vi "PH_SRDG645.PC Write PSDB.vi"(0 "i ref in":refnum<vi>, 5 "error IO":errorcluster) -> (14 "i ref out":refnum<vi>, 19 "error out":errorcluster)   [LabVIEW 2014, in "PH_SRDG645.lvlib"]
doc: "This is the proc case which writes data to the PHELIX shot data base."
uses:
  PH_SRDG645.lvlib
  PH_Basics/PH_PSDBWriter/PH_PSDBWriter.Numeric dataset.ctl
  PH_Basics/PH_PSDBWriter/PH_PSDBWriter.lvlib
  PH_Basics/PH_StatusHandler/PH_StatusHandler.lvlib
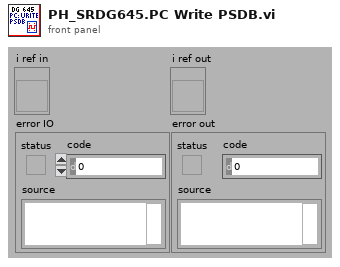
[diagram p1: front panel]
types:
  T1 = typedef "PH_PSDBWriter.lvlib/PH_PSDBWriter.Numeric dataset.ctl" = cluster{"name":string, "data":dbl, "unit":string}
  T2 = typedef "PH_SRDG645.lvlib/PH_SRDG645.i attribute.ctl" = cluster{"GUI Refs":cluster{"Delete":refnum<vi>, "Device Errors":refnum<vi>, "Trigger":refnum<vi>, "Default Name":refnum<vi>, "Firmware Revision":refnum<vi>, "Serial Number":refnum<vi>, "Model":refnum<vi>, "Visa resource name":refnum<vi>}, "Service ID Rate":i32, "Service IDs Channelinfo":i32[], "VISA resource name":refnum<visa-resource-name>, "Device Errors":cluster{"code":i32, "Text":string}[], "Trigger":T3, "Channels":cluster{"T1":T4, "A":T4, "B":T4, "C":T4, "D":T4, "E":T4, "F":T4, "G":T4, "H":T4}, "GUI Refs Channels":refnum<vi>[], "Outputs":cluster{"AB":cluster{"Level Offset [V]":dbl, "Amplitue [V]":dbl, "Polarity":i32}, "CD":cluster{"Level Offset [V]":dbl, "Amplitue [V]":dbl, "Polarity":i32}, "EF":cluster{"Level Offset [V]":dbl, "Amplitue [V]":dbl, "Polarity":i32}, "GH":cluster{"Level Offset [V]":dbl, "Amplitue [V]":dbl, "Polarity":i32}, "T0":cluster{"Level Offset [V]":dbl, "Amplitue [V]":dbl, "Polarity":i32}}, "GUI Refs Outputs":refnum<vi>[], "Serial Number":string, "Firmweare Revision":string, "Model":string}
  T3 = typedef "PH_SRDG645.lvlib/PH_SRDG645.Trigger.ctl" = cluster{"Source":i32, "Rate [Hz]":dbl, "Level [V]":dbl}
  T4 = typedef "PH_SRDG645.lvlib/PH_SRDG645.Channel Settings.ctl" = cluster{"Delay [s]":dbl, "relative to":i32}
  T5 = cluster{"Level Offset [V]":dbl, "Amplitue [V]":dbl, "Polarity":i32}
  T6 = cluster{"Level Offset [V]":dbl, "Amplitue [V]":dbl, "Polarity":i32}[]
  T7 = typedef "PH_PSDBWriter.lvlib/PH_PSDBWriter.String dataset.ctl" = cluster{"name":string, "data":string, "unit":string}
  T8 = typedef "PH_PSDBWriter.lvlib/PH_PSDBWriter.PSDB Dataset.ctl" = cluster{"Version":i32, "2D data Input":T9[], "Boolean Input":T11[], "Image Input":T12[], "Numeric Input":T1[], "String Input":T7[]}
  T9 = typedef "PH_PSDBWriter.lvlib/PH_PSDBWriter.2D dataset.ctl" = cluster{"name":string, "data":dbl[][], "axis description":T10}
  T10 = typedef "PSDB.lvlib/PSDB_AxisDescription.ctl" = cluster{"x axis label":string, "y axis label":string, "x axis unit":string, "y axis unit":string}
  T11 = typedef "PH_PSDBWriter.lvlib/PH_PSDBWriter.Boolean dataset.ctl" = cluster{"name":string, "data":bool, "unit":string}
  T12 = typedef "PH_PSDBWriter.lvlib/PH_PSDBWriter.Image dataset.ctl" = cluster{"name":string, "data":T13, "unit":string}
  T13 = typedef "IMAQ Image.ctl" = refnum<image>
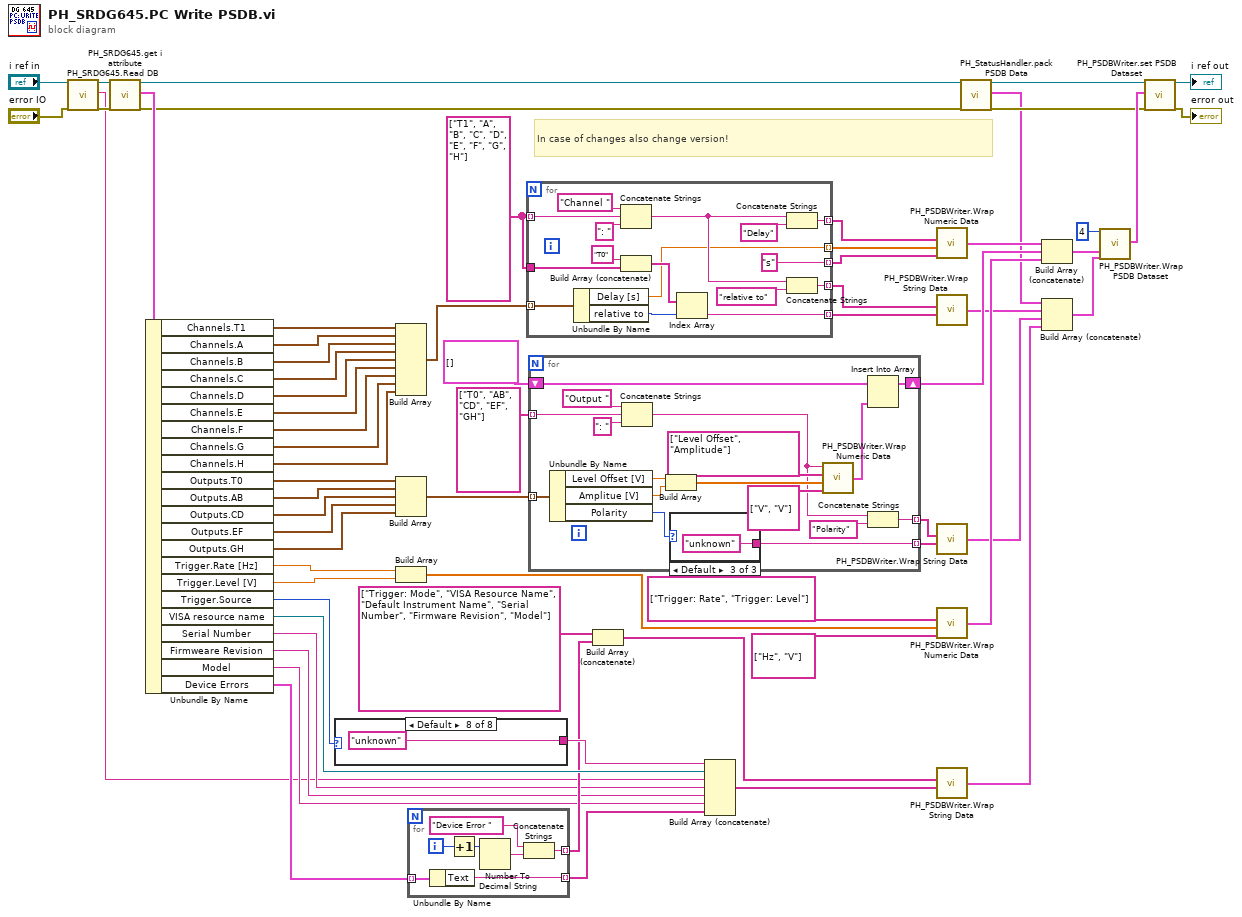
[diagram p0: block diagram]
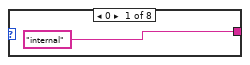
[diagram p2: hidden frame]
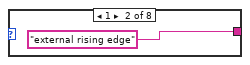
[diagram p3: hidden frame]
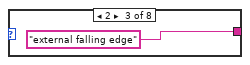
[diagram p4: hidden frame]
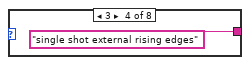
[diagram p5: hidden frame]
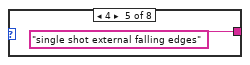
[diagram p6: hidden frame]
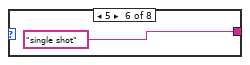
[diagram p7: hidden frame]
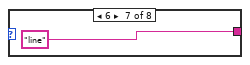
[diagram p8: hidden frame]
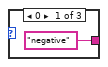
[diagram p9: hidden frame]
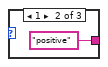
[diagram p10: hidden frame]
diagram:
  w32 = string[] ["T1", "A", "B", "C", "D", "E", "F", "G", "H"]
  # "In case of changes also change version!"
  n1 = call "PH_SRDG645.Read DB.vi"("i ref in"="i ref in", "error in"="error IO") -> ("i ref out"=w15:refnum<vi>, "Default Name"=w14:string, "error out"=w16:errorcluster)  [unwired: 15 in]
  n2 = call "PH_SRDG645.get i attribute.vi"("i ref in"=w15, "error in (no error)"=w16) -> ("i ref out"=w4:refnum<vi>, "i attribute"=w49:T2, "error out"=w5:errorcluster)  [unwired: 15 in]
  n3 = Unbundle By Name(w49) -> ("Channels.T1"=w66:T4, "Channels.A"=w65:T4, "Channels.B"=w64:T4, "Channels.C"=w63:T4, "Channels.D"=w62:T4, "Channels.E"=w37:T4, "Channels.F"=w61:T4, "Channels.G"=w36:T4, "Channels.H"=w35:T4, "Outputs.T0"=w60:T5, "Outputs.AB"=w59:T5, "Outputs.CD"=w58:T5, "Outputs.EF"=w57:T5, "Outputs.GH"=w38:T5, "Trigger.Rate [Hz]"=w42:dbl, "Trigger.Level [V]"=w55:dbl, "Trigger.Source"=w47:i32, "VISA resource name"=w52:refnum<visa-resource-name>, "Serial Number"=w19:string, "Firmweare Revision"=w18:string, "Model"=w17:string, "Device Errors"=w53:cluster{"code":i32, "Text":string}[])
  n4 = case shown="Default" w47 {
    tunnel: ["internal" "external rising edge" "external falling edge" "single shot external rising edges" "single shot external falling edges" "single shot" "line" "unknown"] -> w46
    frame 0 {
    }
    frame 1 {
    }
    frame 2 {
    }
    frame 3 {
    }
    frame 4 {
    }
    frame 5 {
    }
    frame 6 {
    }
    frame Default {
    }
  }
  n5 = Build Array(w66, w65, w64, w63, w62, w37, w61, w36, w35) -> (w26:T4[])
  n6 = Build Array(w60, w59, w58, w57, w38) -> (w56:T6)
  n7 = Build Array(w42, w55) -> (w41:dbl[])
  n8 = for {
    tunnel: w53 -> [w81] mode=indexing
    tunnel: [w80] -> w51 mode=indexing
    tunnel: [w75] -> w44 mode=indexing
    i -> [w79]
    n9 = Unbundle By Name(w81) -> ("Text"=w80:string)
    n10 = Increment(x=w79) -> (x+1=w78:i32)
    n11 = Number To Decimal String(number=w78) -> (decimal integer string=w76:string)  [unwired: 1 in]
    n12 = Concatenate Strings("Device Error ", w76) -> (w75:string)
  }
  n13 = for {
    tunnel: w26 -> [w97] mode=indexing
    tunnel: w32 -> [w94] mode=indexing
    tunnel: w32 -> [w93]
    tunnel: [w89] -> w31 mode=indexing
    tunnel: [w87] -> w30 mode=indexing
    tunnel: ["s" ("string")] -> w28 mode=indexing
    tunnel: [w83] -> w27 mode=indexing
    tunnel: [w82] -> w29 mode=indexing
    n14 = Unbundle By Name(w97) -> ("Delay [s]"=w82:dbl, "relative to"=w90:i32)
    n15 = Concatenate Strings("Channel ", w94, ": " ("string")) -> (w85:string)
    n16 = Build Array (concatenate)("T0", w93) -> (w91:string[])
    n17 = Index Array(array=w91, index=w90) -> (element=w89:string)
    n18 = Concatenate Strings(w85, "Delay" ("string")) -> (w83:string)
    n19 = Concatenate Strings(w85, "relative to" ("string")) -> (w87:string)
  }
  n20 = for {
    tunnel: w56 -> [w114] mode=indexing
    shift-right: [w113] -> w24
    shift-left: T1[] [] -> [w112]
    tunnel: string[] ["T0", "AB", "CD", "EF", "GH"] -> [w106] mode=indexing
    tunnel: [w101] -> w34 mode=indexing
    tunnel: [w98] -> w33 mode=indexing
    n21 = Unbundle By Name(w114) -> ("Level Offset [V]"=w107:dbl, "Amplitue [V]"=w108:dbl, "Polarity"=w102:i32)
    n22 = Concatenate Strings("Output " ("string"), w106, ": " ("string")) -> (w100:string)
    n23 = Build Array(w107, w108) -> (w105:dbl[])
    n24 = case shown="Default" w102 {
      tunnel: ["negative" ("string") "positive" ("string") "unknown" ("string")] -> w101
      frame 0 {
      }
      frame 1 {
      }
      frame Default {
      }
    }
    n25 = call "PH_PSDBWriter.Wrap Numeric Data.vi"("Unit Array"=string[] ["V", "V"], "Data Array"=w105, "Name Array"=string[] ["Level Offset", "Amplitude"], "Name Prefix"=w100) -> ("PSDB Numeric Data Array"=w109:T1[])
    n26 = Insert Into Array(array=w112, new element=w109) -> (w113:T1[])  [unwired: 1 in]
    n27 = Concatenate Strings(w100, "Polarity") -> (w98:string)
  }
  n28 = Build Array (concatenate)(string[] ["Trigger: Mode", "VISA Resource Name", "Default Instrument Name", "Serial Number", "Firmware Revision", "Model"], w44) -> (w43:string[])
  n29 = Build Array (concatenate)(w46, w52, w14, w19, w18, w17, w51) -> (w48:string[])
  n30 = call "PH_PSDBWriter.Wrap Numeric Data.vi"("Unit Array"=w28, "Data Array"=w29, "Name Array"=w27) -> ("PSDB Numeric Data Array"=w25:T1[])  [unwired: 1 in]
  n31 = call "PH_PSDBWriter.Wrap String Data.vi"("Data Array"=w31, "Name Array"=w30) -> ("PSDB String Data Array"=w22:T7[])  [unwired: 2 in]
  n32 = call "PH_PSDBWriter.Wrap String Data.vi"("Data Array"=w34, "Name Array"=w33) -> ("PSDB String Data Array"=w21:T7[])  [unwired: 2 in]
  n33 = call "PH_PSDBWriter.Wrap Numeric Data.vi"("Unit Array"=string[] ["Hz", "V"], "Data Array"=w41, "Name Array"=string[] ["Trigger: Rate", "Trigger: Level"]) -> ("PSDB Numeric Data Array"=w23:T1[])  [unwired: 1 in]
  n34 = call "PH_PSDBWriter.Wrap String Data.vi"("Data Array"=w48, "Name Array"=w43) -> ("PSDB String Data Array"=w20:T7[])  [unwired: 2 in]
  n35 = call "PH_StatusHandler.pack PSDB Data.vi"("VI in"=w4, "error in (no error)"=w5) -> ("VI out"=w2:refnum<vi>, "PSDB String Data Array"=w1:T7[], "error out"=w3:errorcluster)  [unwired: 15 in]
  n36 = Build Array (concatenate)(w25, w24, w23) -> (w11:T1[])
  n37 = Build Array (concatenate)(w1, w22, w21, w20) -> (w10:T7[])
  n38 = call "PH_PSDBWriter.Wrap PSDB Dataset.vi"("Version"=4, "Numeric Input"=w11, "String Input"=w10) -> ("PSDB Dataset"=w8:T8)  [unwired: 16 in]
  n39 = call "PH_PSDBWriter.set PSDB Dataset.vi"("VI in"=w2, "PSDB Dataset"=w8, "error in (no error)"=w3) -> ("VI out"=→"i ref out":refnum<vi>, "error out"=→"error out":errorcluster)  [unwired: 15 in]
